vi "Read Tag Element (Direction).vi"(8 "error in":errorcluster, 9 "default":T1, 10 "Tag Name":string, 11 "node in":refnum<k20>) -> (0 "error out":errorcluster, 1 "value":T1, 3 "node out":refnum<k20>)   [LabVIEW 2020, in "ARINC 429 Import.lvlib"]
uses:
  ARINC 429 Import.lvlib
  Shared/Direction.ctl
  <resource>/objmgr/DOMUserDefRef.rc
  <vilib>/xml/NI_XML.lvlib
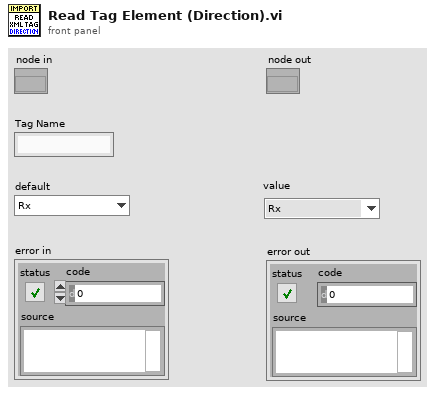
[diagram p1: front panel]
types:
  T1 = typedef "Direction.ctl" = enum16{"Rx", "Tx"}
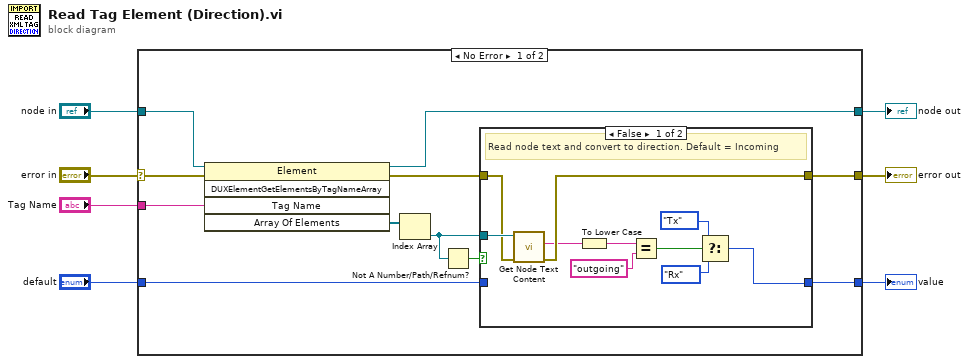
[diagram p0: block diagram]
diagram:
  n1 = case shown="No Error" "error in" {
    selector: "error in" -> [w8 w33]
    tunnel: [w18 w33] -> w7
    tunnel: "node in" -> [w14 w32]
    tunnel: "Tag Name" -> [w12 _]
    tunnel: [w11 w31] -> w4
    tunnel: [w10 w32] -> w3
    tunnel: "default" -> [w9 w31]
    frame No Error {
      n2 = invoke class="Element" method="DUXElementGetElementsByTagNameArray"(reference=w14, error in=w8, "Tag Name"=w12) -> (reference out=w10:refnum<k20>, error out=w17:errorcluster, "Array Of Elements"=w13:refnum<k20>[])  [unwired: 2 in, 2 out]
      n3 = Index Array(array=w13) -> (element=w15:refnum<k20>)  [unwired: 1 in]
      n4 = Not A Number/Path/Refnum?(number/path/refnum=w15) -> (NaN/Path/Refnum?=w16:bool)
      n5 = case shown="False" w16 {
        tunnel: w15 -> [w28 _]
        tunnel: w17 -> [w27 w30]
        tunnel: [w19 w29] -> w11
        tunnel: [w26 w30] -> w18
        tunnel: w9 -> [_ w29]
        frame False {
          # "Read node text and convert to direction. Default = Incoming"
          n6 = call <vilib>:"Get Node Text Content.vi"("error in (no error)"=w27, "node in"=w28) -> ("error out"=w26:errorcluster, "node text"=w25:string)  [unwired: 7 in, 1 out]
          n7 = To Lower Case(string=w25) -> (all lower case string=w24:string)
          n8 = Equal?(x=w24, y="outgoing") -> (x = y?=w22:bool)
          n9 = Select(t=Direction."Tx" ("default"), s=w22, f=Direction."Rx" ("default")) -> (s? t:f=w19:T1)
        }
        frame True {
          # "pass default if element doesn't exist"
        }
      }
    }
    frame Error {
    }
  }
  "error out" <- w7
  "node out" <- w3
  "value" <- w4
